vi "ImagesGetIvsP.vi"(8 "error in (no error)":errorcluster, 11 "Image in":refnum<class "Image.lvclass">) -> (0 "error out":errorcluster, 1 "Added Image Intensity (I_new)":dbl[](array[numeric]), 2 "Intensity vs Stage Position (mm)":cluster{dbl[], dbl[]}[](array[cluster]), 3 "Image out":refnum<class "Image.lvclass">)   [LabVIEW 2012, in "Image.lvclass"]
doc: "Saves image based on array data\nEdit for grab scan mode"
uses:
  classes/Image.lvclass
  classes/Image.lvclass/Image.ctl
  ImageIvsPProcess2D.vi
  ImageIvsPProcessPS.vi
  ImageIvsPProcessPSTime.vi
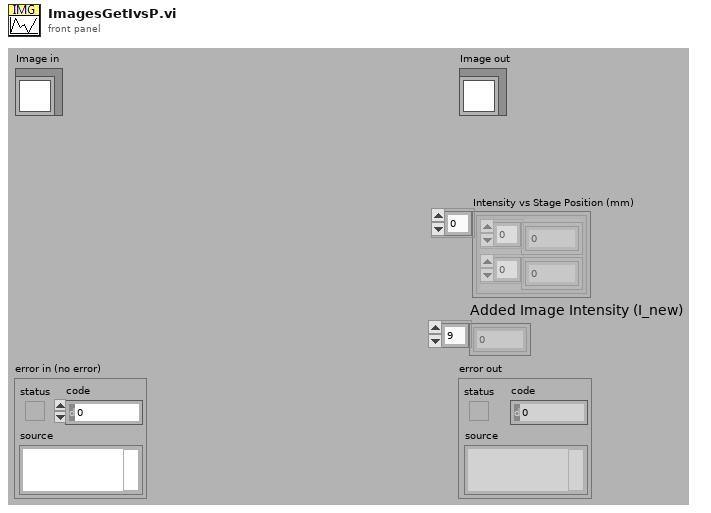
[diagram p1: front panel]
types:
  T1 = typedef "ScanMode.ctl" = enum16{"None", "Continuous", "Point Scan (CH3 cursor)", "Point Scan Move (CH3 cursor)", "Grab", "Grab Move Stage", "Grab Move Z-stage", "Cont. Move Z-stage", "Spec Move Stage", "Spec Move Cont", "Surf Calib"}
  T2 = cluster{"Stage Position (mm)":dbl[], "Image intensity":dbl[]}[]
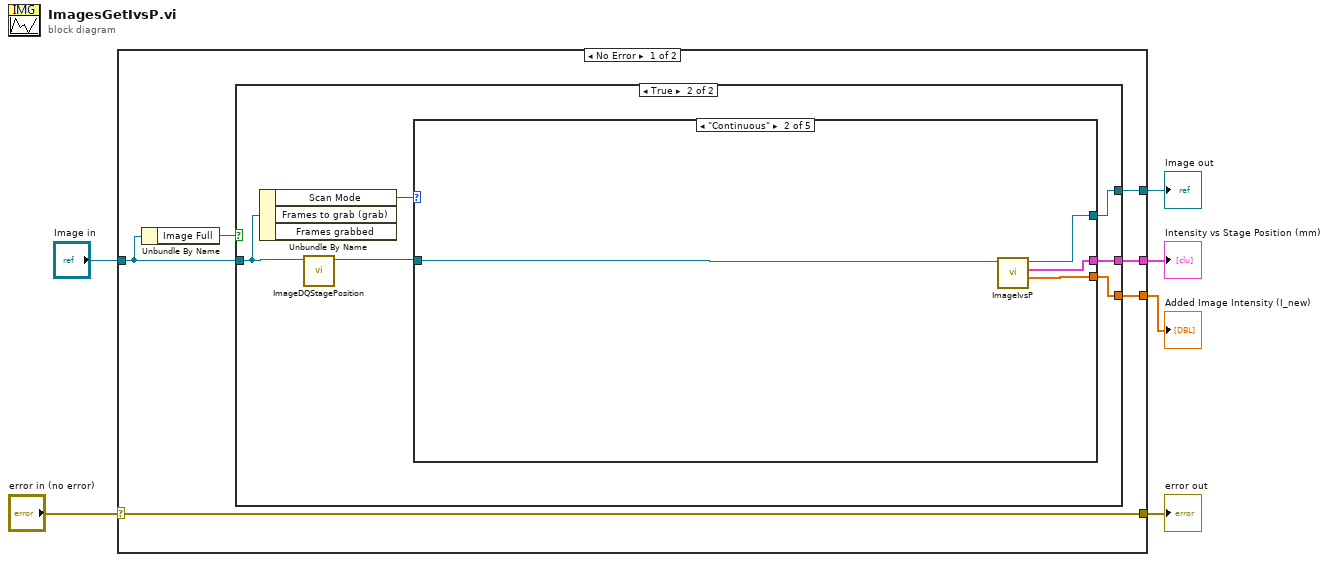
[diagram p0: block diagram]
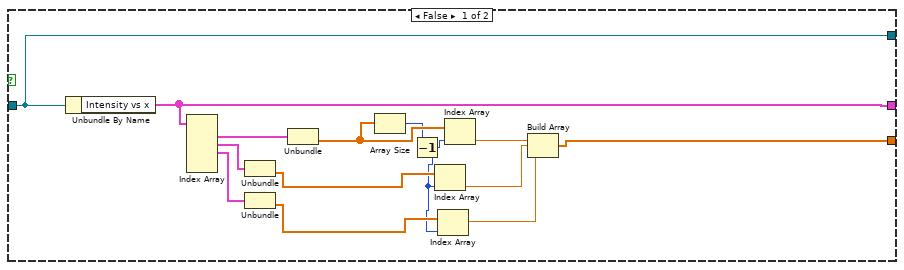
[diagram p2: hidden frame]
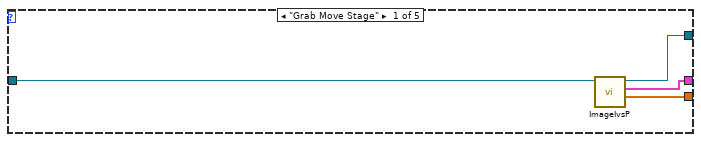
[diagram p3: hidden frame]
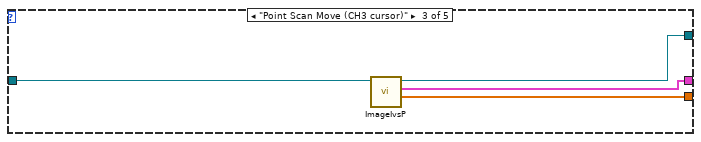
[diagram p4: hidden frame]
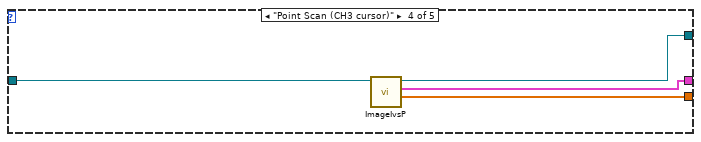
[diagram p5: hidden frame]
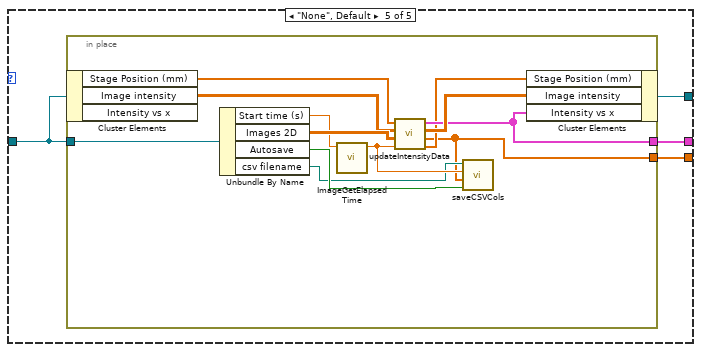
[diagram p6: hidden frame]
diagram:
  n1 = case shown="No Error" "error in (no error)" {
    selector: "error in (no error)" -> [w12 w66]
    tunnel: [w12 w66] -> w5
    tunnel: [w11 w65] -> w4
    tunnel: "Image in" -> [w10 w65]
    tunnel: [w8 _] -> w2
    tunnel: [w7 _] -> w1
    frame No Error {
      n2 = Unbundle By Name(w10) -> ("Image Full"=w9:bool)
      n3 = case shown="True" w9 {
        tunnel: [w26 w32] -> w11
        tunnel: w10 -> [w26 w28]
        tunnel: [w25 w30] -> w8
        tunnel: [w15 w29] -> w7
        frame False {
          n4 = Unbundle By Name(w26) -> ("Intensity vs x"=w25:cluster{dbl[], dbl[]}[])
          n5 = Index Array(array=w25) -> (element #1=w24:cluster{dbl[], dbl[]}, element #2=w23:cluster{dbl[], dbl[]}, element #3=w22:cluster{dbl[], dbl[]})  [unwired: 5 in, 2 out]
          n6 = Unbundle(w23) -> (w20:dbl[])  [unwired: 1 out]
          n7 = Unbundle(w22) -> (w19:dbl[])  [unwired: 1 out]
          n8 = Unbundle(w24) -> (w21:dbl[])  [unwired: 1 out]
          n9 = Array Size(array=w21) -> (size(s)=w14:i32)
          n10 = Decrement(x=w14) -> (x-1=w13:i32)
          n11 = Index Array(array=w20, index=w13) -> (element=w18:dbl)
          n12 = Index Array(array=w19, index=w13) -> (element=w17:dbl)
          n13 = Index Array(array=w21, index=w13) -> (element=w16:dbl)
          n14 = Build Array(w16, w18, w17) -> (w15:dbl[])
        }
        frame True {
          n15 = Unbundle By Name(w28) -> ("Scan Mode"=w31:T1)  [unwired: 2 out]
          n16 = call "ImageDQStagePosition.vi"("Image in"=w28) -> ("Image out"=w27:refnum<class "Image.lvclass">)  [unwired: 10 in]
          n17 = case shown="\"Continuous\"" w31 {
            tunnel: [w34 w38 w42 w46 w52] -> w30
            tunnel: w27 -> [w36 w40 w44 w48 w51]
            tunnel: [w35 w39 w43 w47 w50] -> w32
            tunnel: [w33 w37 w41 w45 w49] -> w29
            frame "Grab Move Stage" {
              n18 = call-poly "ImageIvsP.vi"("Image in"=w36) -> ("Added Image Intensity (I_new)"=w33:dbl[], "Array"=w34:T2, "Image out"=w35:refnum<class "Image.lvclass">)  [unwired: 8 in]
            }
            frame "Continuous" {
              n19 = call-poly "ImageIvsP.vi"("Image in"=w40) -> ("Added Image Intensity (I_new)"=w37:dbl[], "Array"=w38:T2, "Image out"=w39:refnum<class "Image.lvclass">)  [unwired: 8 in]
            }
            frame "Point Scan Move (CH3 cursor)" {
              n20 = call-poly "ImageIvsP.vi"("Image in"=w44) -> ("Added Image Intensity (I_new)"=w41:dbl[], "Array"=w42:T2, "Image out"=w43:refnum<class "Image.lvclass">)  [unwired: 8 in]
            }
            frame "Point Scan (CH3 cursor)" {
              n21 = call-poly "ImageIvsP.vi"("Image in"=w48) -> ("Added Image Intensity (I_new)"=w45:dbl[], "Array"=w46:T2, "Image out"=w47:refnum<class "Image.lvclass">)  [unwired: 8 in]
            }
            frame "None", Default {
              n22 = in-place {
                in-place-border: w51 -> [w64]
                in-place-border: [w60] -> w52
                in-place-border: [w53] -> w49
                n23 = in-place-cluster #1(w51) -> ("Stage Position (mm)"=w55:dbl[], "Image intensity"=w62:dbl[][])  [unwired: 1 out]
                n24 = Unbundle By Name(w64) -> ("Start time (s)"=w58:dbl, "Images 2D"=w63:dbl[][][], "Autosave"=w59:bool, "csv filename"=w54:path)
                n25 = call "ImageGetElapsedTime.vi"("start time"=w58) -> ("time elapsed (s)"=w57:dbl)  [unwired: 10 in]
                n26 = call "updateIntensityData.vi"("new x"=w57, "Images 2D"=w63, "Image Intensity (initial)"=w62, "x-axis (initial)"=w55) -> ("x-axis (final = initial + new)"=w56:dbl[], "Added Image Intensity (I_new)"=w53:dbl[], "Image Intensity (final = I_initial + I_new)"=w61:dbl[][], "Image Intensity vs x"=w60:cluster{dbl[], dbl[]}[])  [unwired: 4 in]
                n27 = call "saveCSVCols.vi"("Autosave"=w59, "y values"=w53, "x"=w57, "Image filename"=w54) -> ()  [unwired: 8 in]
                n28 = in-place-cluster #1("Stage Position (mm)"=w56, "Image intensity"=w61, "Intensity vs x"=w60) -> (w50:refnum<class "Image.lvclass">)
              }
            }
          }
        }
      }
    }
    frame Error {
    }
  }
  "error out" <- w5
  "Image out" <- w4
  "Intensity vs Stage Position (mm)" <- w2
  "Added Image Intensity (I_new)" <- w1
